vi "TCSPC Initialize.vi"(10 "ADC Resolution [exponent]":T1=10 items=["-1"=-1, "1"=0, "4"=2, "16"=4, "64"=6, "256"=8, "1024"=10, "4096"=12]) -> (0 "Error Out":errorcluster, 1 "Page":i32, 2 "Module No":i16, 3 "DLL Path":path, 6 "Serial Number":string[](array[string])=["3F0668", "3F0848"], 7 "SPCMemConfig":T2={"Max Block No"=0, "Blocks Per Frame"=0, "Frames Per Page"=1, "Maxpage"=1, "Block Length"=1} {"Frames Per Page" min=1 step=1; "Maxpage" min=1; "Blocks Per Frame" min=1 step=1})   [LabVIEW 2023]
doc: "This example demonstrates how to use the Becker & Hickl LabVIEW wrapper VIs to acquire one single decay curve from one SPC module.\n\ninfo@becker-hickl.com"
uses:
  Drivers/BH TCSPC/SPC_Wrappers/SPC_Controls/ConfigMem.ctl
  Drivers/BH TCSPC/SPC_Wrappers/SPC_Controls/ADCResolution.ctl
  Drivers/BH TCSPC/SPC_Wrappers/SPC_Controls/par_id.ctl
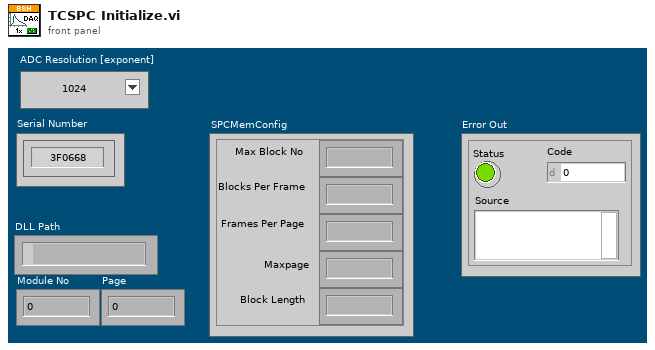
[diagram p1: front panel]
types:
  T1 = typedef "ADCResolution.ctl" = i16
  T2 = typedef "ConfigMem.ctl" = cluster{"Max Block No":i32, "Blocks Per Frame":i32, "Frames Per Page":i32, "Maxpage":i32, "Block Length":i32}
  T3 = typedef "par_id.ctl" = i16
  T4 = typedef "SPCModInfo.ctl" = cluster{"Module Type":T5, "Bus Number":i16, "Slot Number":i16, "in Use":i16, "Init Status":i16, "Base I/O Addr":u16}
  T5 = typedef "ModuleType.ctl" = i16
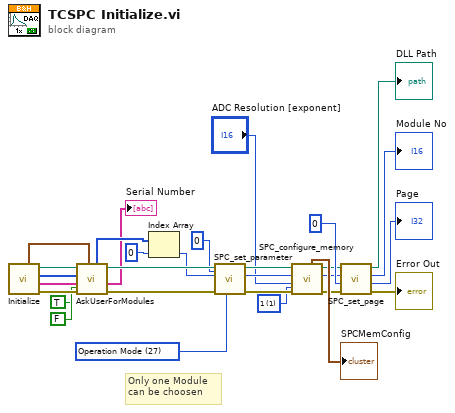
[diagram p0: block diagram]
diagram:
  w15 = i16 1 items=["1"=1, "2"=2, "3"=3, "4"=4, "5"=5, "6"=6, "7"=7, "8"=8, "9"=9, "10"=10, "11"=11, "12"=12, "13"=13, "14"=14, "15"=15, "16"=16] ("No of Routing\nChannels")
  w19 = T3 27 items=["CFD Limit Low", "CFD Limit High", "CFD Zero Cross Level", "CFD Holdoff", "SYNC Zero Cross Level", "SYNC Freq Divider", "SYNC Holdoff", "SYNC Threshold", "TAC Range", "TAC Gain", "TAC Offset", "TAC Limit Low", "TAC Limit High", "ADC Resolution", "External Latch Delay", "Collect Time", "Display Time", "Repeat Time", "Stop On Time", "Stop On Overflow", "Dither Range", "Count Increment", "Memory Bank", "Dead Time Compensation", "Scan Control", "Routing Mode", "TAC Enable Hold", "Operation Mode", "Scan Size X", "Scan Size Y", "Scan Routing X Bits", "Scan Routing Y Bits", "Scan Polarity", "Scan Flyback", "Scan Borders", "Pixel Time", "Pixel Clock Source", "Scan Line Compression", "External Trigger Condition", "External Pixel Clock Divider", "Rate Counting Time", "Macro Time Clock", "ADD Signal Source", "ADC Zoom", "XY Gain", "Image Size X", "Image Size Y", "Image Routing X Bits", "Image Routing Y Bits", "Master Clock", "ADC Sample Delay", "Detector Type", "X Axis Type", "Channel Enable", "Channel Slope", "Channel Spec_no"] ("SPC parameter ID")
  # "Only one Module\ncan be choosen"
  n1 = call "Initialize.vi"() -> ("ErrorOut"=w28:errorcluster, "SerialNumbersArray"=w26:string[], "ModuleNoArray"=w25:i16[], "DLL Path"=w29:path, "SPCModulesArray"=w27:T4[])  [unwired: 7 in]
  n2 = call "AskUserForModules.vi"("MultiModule"=FALSE, "SkipDialog"=TRUE, "SPCModulesArray"=w27, "Error In"=w28, "Serial Number"=w26, "ModuleNoArray"=w25, "DLL Path"=w29) -> ("Error Out"=w21:errorcluster, "ActiveSerialNumbers"=→"Serial Number":string[], "DLL Path"=w22:path, "ActiveModuleNo"=w24:i16[])  [unwired: 1 out]
  n3 = Index Array(array=w24, index=0) -> (element=w18:i16)
  n4 = call "SPC_set_parameter.vi"("SPC parameter ID"=w19, "Parameter Value"=u16 0 ("Operation Mode"), "Error In"=w21, "Module no"=w18, "DLL Path"=w22) -> ("Error Out"=w16:errorcluster, "Module no"=w14:i16, "DLL Path"=w17:path)  [unwired: 3 in, 1 out]
  n5 = call "SPC_configure_memory.vi"("No of Routing\nChannels"=w15, "Error In"=w16, "ADC Resolution [exponent]"="ADC Resolution [exponent]", "Module No"=w14, "DLL Path"=w17) -> ("Error Out"=w11:errorcluster, "Module No"=w9:i16, "DLL Path"=w10:path, "SPCMemConfig"=→"SPCMemConfig":T2)  [unwired: 2 in, 1 out]
  n6 = call "SPC_set_page.vi"("Error In"=w11, "Page"=0 ("ADC resolution"), "Module No"=w9, "DLL Path"=w10) -> ("Error Out"=→"Error Out":errorcluster, "Page"=→"Page":i32, "Module No"=→"Module No":i16, "DLL Path"=→"DLL Path":path)  [unwired: 4 in]
